vi "exec.vi"(8 "error in (no error)":errorcluster, 10 "context":refnum<class "Context.lvclass">, 11 "SwitchToStreamMode in":refnum<class "SwitchToStreamMode.lvclass">) -> (0 "error out":errorcluster, 2 "context 2":refnum<class "Context.lvclass">, 3 "SwitchToStreamMode out":refnum<class "SwitchToStreamMode.lvclass">)   [LabVIEW 2013, in "SwitchToStreamMode.lvclass"]
uses:
  SwitchToStreamMode.lvclass
  Context/Context.lvclass
  SwitchToStreamMode.lvclass/SwitchToStreamMode.ctl
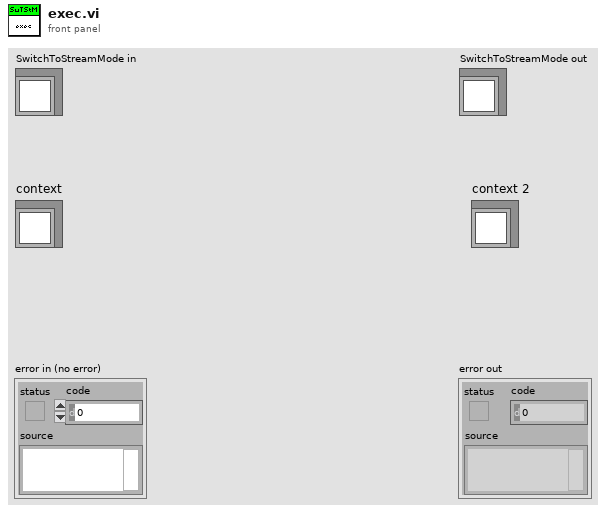
[diagram p1: front panel]
types:
  T1 = typedef "Stream Mode Algorithm.ctl" = enum16{"FrontPanelValuesDirectly"}
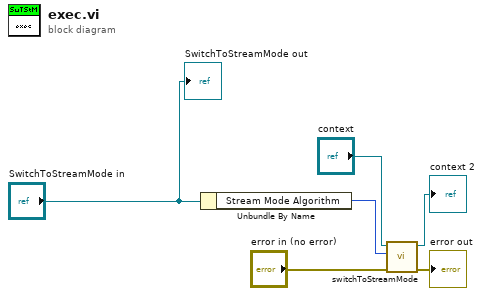
[diagram p0: block diagram]
diagram:
  n1 = Unbundle By Name("SwitchToStreamMode in") -> ("Stream Mode Algorithm"=w1:T1)
  n2 = call "switchToStreamMode.vi"("error in (no error)"="error in (no error)", "Stream Mode Algorithm"=w1, "Context in"="context") -> ("error out"=→"error out":errorcluster, "Context out"=→"context 2":refnum<class "Context.lvclass">)  [unwired: 7 in]
  "SwitchToStreamMode out" <- "SwitchToStreamMode in"
